vi "Get Projects available.vi"() -> (3 "Projects Available":string[](array[string]))   [LabVIEW 2020, in "Panter Dashboard.lvlib"]
uses:
  Panter Dashboard.lvlib
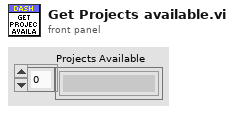
[diagram p1: front panel]
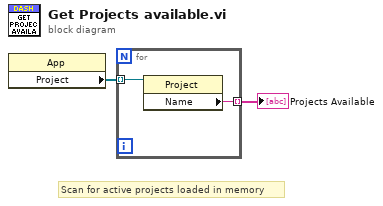
[diagram p0: block diagram]
diagram:
  # "Scan for active projects loaded in memory"
  n1 = property class="App"() -> ("Project"=w1:refnum<vi>[])  [unwired: 2 in, 2 out]
  n2 = for {
    tunnel: w1 -> [w4] mode=indexing
    tunnel: [w3] -> w2 mode=indexing
    n3 = property class="Project"(reference=w4) -> ("Name"=w3:string)  [unwired: 1 in, 2 out]
  }
  "Projects Available" <- w2
